vi "Single VLC DisplayN.vi"() -> ()   [LabVIEW 2017]
uses:
  <vilib>/Utility/miscctls.llb/LVRectTypeDef.ctl
  VideoWindowsCommand.ctl
  Video Command type.ctl
  <vilib>/Utility/config.llb/NI_LVConfig.lvlib
  System.Windows.Forms
panel:
  in  "Camera 1":refnum<k24>(container)
  in  "Hide":bool
  in  "Connect":bool
  in  "Cameras":string[](array[string])=["http://admin:pass1234@192.168.1.64/ISAPI/Streaming/channels/102/httpPreview", "http://admin:pass1234@192.168.1.65/ISAPI/Streaming/channels/102/httpPreview", "//192.168.1.119:4747/video"]
  in  "Address":string
  out "InstanceNumber":i32
  in  "Video Feed":enum16{"Camera 1", "Camera2", "Mobile"}(ring)=enum."Camera2"
  in  "Exit":bool
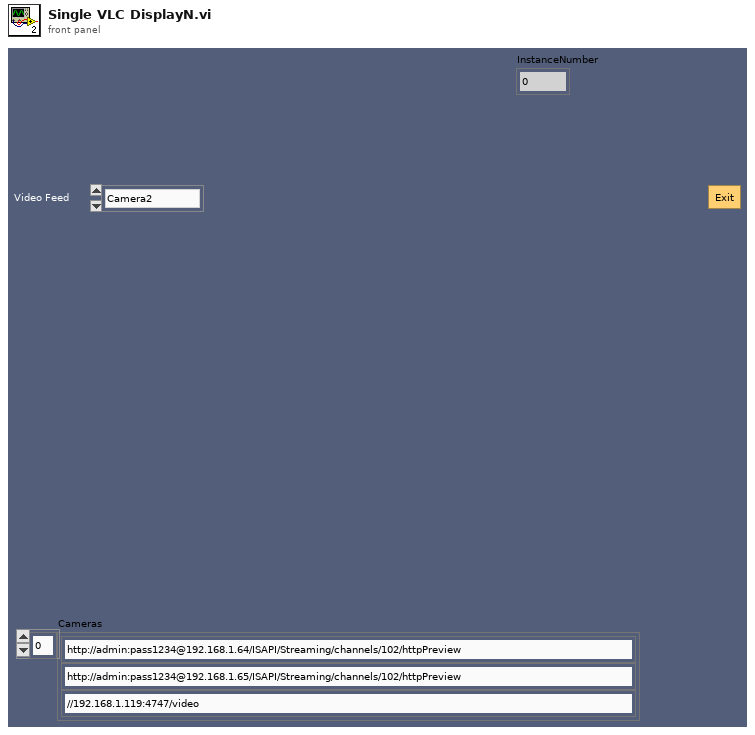
[diagram p1: front panel]
types:
  T1 = typedef "LVRectTypeDef.ctl" = cluster{"Left":i16, "Top":i16, "Right":i16, "Bottom":i16}
  T2 = typedef "NI_LVConfig.lvlib/Config Data RefNum.ctl" = refnum<k1>
  T3 = typedef "VideoWindowsCommand.ctl" = cluster{"Position":cluster{"Right":i32, "Bottom":i32}, "Action":T4, "Camera Addresses":cluster{"Camera 1":string, "Camera 2":string, "Mobile":string}}
  T4 = typedef "Video Command type.ctl" = enum16{"Show", "Hide", "Exit", "Kick"}
  T5 = cluster{"Camera 1":string, "Camera 2":string, "Mobile":string}
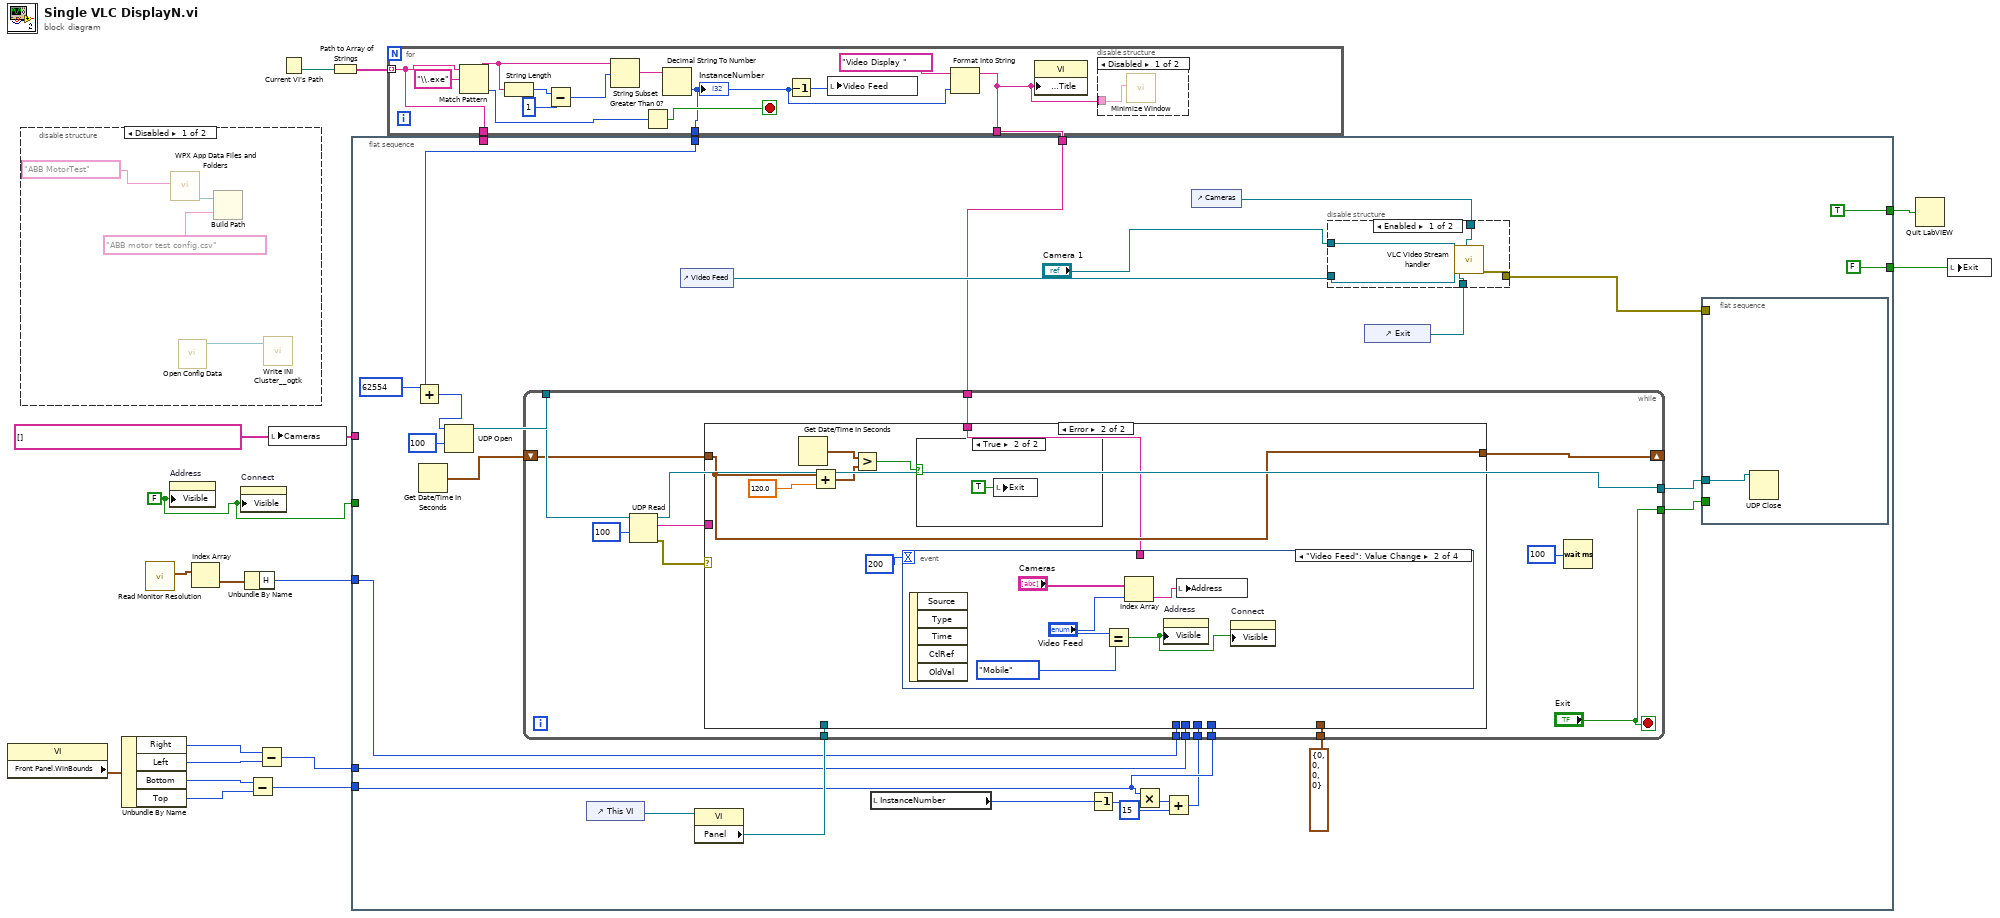
[diagram p0: block diagram]
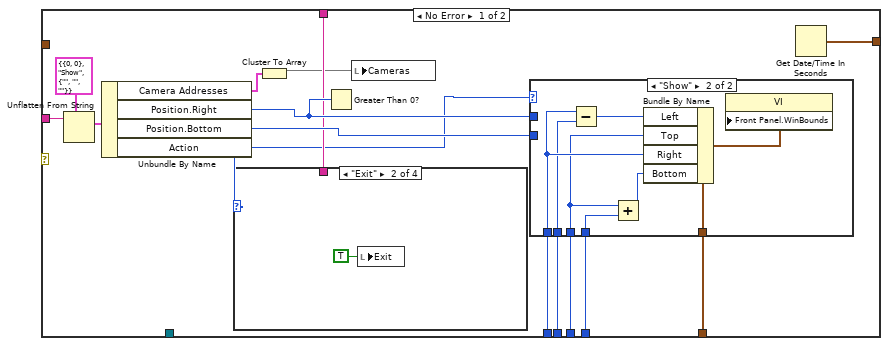
[diagram p4: hidden frame]
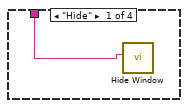
[diagram p5: hidden frame]
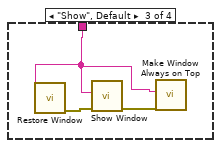
[diagram p6: hidden frame]
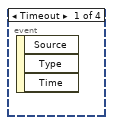
[diagram p10: hidden frame]
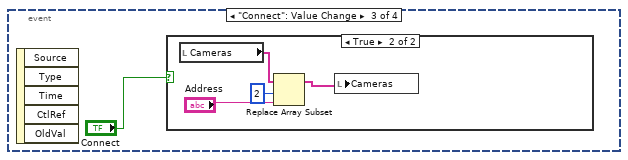
[diagram p11: hidden frame]
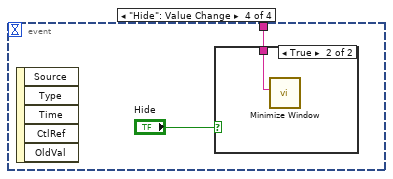
[diagram p13: hidden frame]
diagram:
  w1 = string[] [] ("Cameras")
  w4 = FALSE ("Visible")
  n1 = property class="VI"() -> ("Front Panel.WinBounds"=w12:T1)  [unwired: 2 in, 2 out]
  n2 = disable-structure shown="Disabled" {
    frame Disabled {
      n3 = call "WPX App Data Files and Folders.vi"("ApplicationName"="ABB MotorTest") -> ("DataFolder"=w20:path)  [unwired: 7 in, 3 out]
      n4 = call <vilib>:"Open Config Data.vi"() -> ("refnum"=w23:T2)  [unwired: 9 in, 2 out]
      n5 = Build Path(base path=w20, name or relative path="ABB motor test config.csv") -> ()  [unwired: 1 out]
      n6 = call <userlib>:"Write INI Cluster__ogtk.vi"("refnum"=w23) -> ()  [unwired: 9 in, 2 out]
    }
    frame Enabled {
    }
  }
  n7 = Unbundle By Name(w12) -> ("Right"=w9:i16, "Left"=w8:i16, "Bottom"=w11:i16, "Top"=w10:i16)
  n8 = call "Read Monitor Resolution.vi"() -> ("Monitor Resolution"=w14:cluster{"V":i16, "H":i16}[])  [unwired: 9 in, 2 out]
  n9 = property on="Address" class="Str"("Visible"=w4) -> ()  [unwired: 2 in, 2 out]
  n10 = Index Array(array=w14) -> (element=w13:cluster{"V":i16, "H":i16})  [unwired: 1 in]
  n11 = property on="Connect" class="Bool"("Visible"=w4) -> ()  [unwired: 2 in, 2 out]
  n12 = Unbundle By Name(w13) -> ("H"=w7:i16)
  n13 = Subtract(x=w11, y=w10) -> (x-y=w5:i16)
  n14 = Subtract(x=w9, y=w8) -> (x-y=w6:i16)
  n15 = local write "Cameras"(w1) -> ()
  n16 = Current VI's Path() -> (path=w19:path)
  n17 = Path to Array of Strings(0:w19) -> (2:w18:string[])  [unwired: 1 out]
  n18 = flat-sequence {
    tunnel: w17 -> [w40]
    tunnel: w16 -> [_]
    tunnel: w15 -> [w38]
    tunnel: w7 -> [w37]
    tunnel: w6 -> [w36]
    tunnel: w5 -> [w32]
    tunnel: w4 -> [_]
    tunnel: [TRUE] -> w3
    tunnel: [FALSE ("Exit")] -> w2
    tunnel: w1 -> [_]
    frame #0 {
      n19 = Add(x=w40, y=u16 62554 ("port")) -> (x+y=w39:i32)
      n20 = Get Date/Time In Seconds() -> (seconds since 1Jan1904=w25:timestamp)
      n21 = UDP Open(9:100 ("timeout ms (25000)"), 11:w39) -> (port=w47:refnum<k16>)  [unwired: 3 in, 2 out]
      n22 = control-ref of="This VI"() -> (w46:refnum<vi>)
      n23 = control-ref of="Video Feed"() -> (w50:refnum<vi>)
      n24 = property class="VI"(reference=w46) -> ("Panel"=w45:refnum<vi>)  [unwired: 1 in, 2 out]
      n25 = local read "InstanceNumber"() -> (w34:i32)
      n26 = Decrement(x=w34) -> (x-1=w33:i32)
      n27 = Multiply(x=w32, y=w33) -> (x*y=w30:i32)
      n28 = Add(x=w30, y=15) -> (x+y=w29:i32)
      n29 = while {
        tunnel: ["Exit"] -> w48
        tunnel: w47 -> [w66]
        tunnel: w45 -> [w62]
        tunnel: [w61] -> w44
        tunnel: w38 -> [w60]
        tunnel: w37 -> [w59]
        tunnel: w36 -> [w58]
        tunnel: T1 {"Left"=0, "Top"=0, "Right"=0, "Bottom"=0} ("Front Panel Window:Window Bounds") -> [w57]
        tunnel: w29 -> [w56]
        tunnel: w32 -> [w55]
        shift-right: [w53] -> _
        shift-left: w25 -> [w52]
        stop <- "Exit" stop-if-true
        n30 = UDP Read(connection ID=w66, timeout ms (25000)=100) -> (data out=w63:string, error out=w64:errorcluster, 3:w61:refnum<k16>)  [unwired: 2 in, 2 out]
        n31 = case shown="Error" w64 {
          tunnel: w63 -> [w82 _]
          tunnel: w62 -> [_ _]
          tunnel: w60 -> [w72 w96]
          tunnel: w59 -> [w77 _]
          tunnel: w58 -> [w76 _]
          tunnel: w57 -> [w75 _]
          tunnel: w56 -> [w74 _]
          tunnel: w55 -> [w73 _]
          tunnel: [w70 w97] -> w53
          tunnel: w52 -> [_ w97]
          frame No Error {
            n32 = Unflatten From String(type=T3 {"Position"={"Right"=0, "Bottom"=0}, "Action"=enum."Show", "Camera Addresses"={"Camera 1"="", "Camera 2"="", "Mobile"=""}}, binary string=w82) -> (value=w80:T3)  [unwired: 3 in, 2 out]
            n33 = Unbundle By Name(w80) -> ("Camera Addresses"=w69:T5, "Position.Right"=w78:i32, "Position.Bottom"=w79:i32, "Action"=w71:T4)
            n34 = case shown="\"Exit\"" w71 {
              tunnel: w72 -> [w83 _ w86 _]
              frame "Hide" {
                n35 = call "Hide Window.vi"("window name (\"\")"=w83) -> ()  [unwired: 5 in, 2 out]
              }
              frame "Exit" {
                n36 = local write "Exit"(TRUE ("Exit")) -> ()
              }
              frame "Show", Default {
                n37 = call "Restore Window.vi"("window name  (\"\")"=w86) -> ("error out"=w85:errorcluster)  [unwired: 5 in, 1 out]
                n38 = call "Show Window.vi"("error in (no error)"=w85, "window name (\"\")"=w86) -> ("error out"=w87:errorcluster)  [unwired: 4 in, 1 out]
                n39 = call "Make Window Always on Top.vi"("error in (no error)"=w87, "window name (\"\")"=w86) -> ()  [unwired: 4 in, 2 out]
              }
              frame "Kick" {
              }
            }
            n40 = Cluster To Array(cluster=w69) -> (array=w68:string[])
            n41 = Greater Than 0?(x=w78) -> ()  [unwired: 1 out]
            n42 = local write "Cameras"(w68) -> ()
            n43 = case shown="\"Show\"" w71 {
              tunnel: w79 -> [_ _]
              tunnel: w78 -> [_ _]
              tunnel: w77 -> [_ w92]
              tunnel: w76 -> [_ w91]
              tunnel: w75 -> [_ w90]
              tunnel: w74 -> [_ w89]
              tunnel: w73 -> [_ w88]
              frame "Hide", Default {
              }
              frame "Show" {
                n44 = Subtract(x=w92, y=w91) -> (x-y=w94:i16)
                n45 = Add(x=w89, y=w88) -> (x+y=w93:i32)
                n46 = Bundle By Name(cluster=w90, "Left"=w94, "Top"=w89, "Right"=w92, "Bottom"=w93) -> (w95:T1)
                n47 = property class="VI"("Front Panel.WinBounds"=w95) -> ()  [unwired: 2 in, 2 out]
              }
            }
            n48 = Get Date/Time In Seconds() -> (seconds since 1Jan1904=w70:timestamp)
          }
          frame Error {
            n49 = Get Date/Time In Seconds() -> (seconds since 1Jan1904=w101:timestamp)
            n50 = Add(x=w97, y=120.0) -> (x+y=w99:timestamp)
            n51 = Greater?(x=w101, y=w99) -> (0:w98:bool)
            n52 = event shown="[1] \"Video Feed\": Value Change" {
              selector: _ -> [_ _ _ _]
              dyn-events: _ -> [_ _ _ _]
              timeout: 200 -> [_ _ _ _]
              tunnel: w96 -> [_ _ _ w114]
              event Timeout {
                n53 = event-data() -> ()  [unwired: 1 in, 3 out]
              }
              event "Video Feed": Value Change {
                n54 = event-data() -> ()  [unwired: 1 in, 5 out]
                n55 = Equal?(x="Video Feed", y=enum16{"Camera 1", "Camera2", "Mobile"}."Mobile") -> (x = y?=w107:bool)
                n56 = Index Array(array="Cameras", index="Video Feed") -> (element=w104:string)
                n57 = property on="Address" class="Str"("Visible"=w107) -> ()  [unwired: 2 in, 2 out]
                n58 = local write "Address"(w104) -> ()
                n59 = property on="Connect" class="Bool"("Visible"=w107) -> ()  [unwired: 2 in, 2 out]
              }
              event "Connect": Value Change {
                n60 = event-data() -> ()  [unwired: 1 in, 5 out]
                n61 = case shown="True" "Connect" {
                  frame False {
                  }
                  frame True {
                    n62 = local read "Cameras"() -> (w113:string[])
                    n63 = Replace Array Subset(array=w113, new element="Address", index=2) -> (w112:string[])
                    n64 = local write "Cameras"(w112) -> ()
                  }
                }
              }
              event "Hide": Value Change {
                n65 = event-data() -> ()  [unwired: 1 in, 5 out]
                n66 = case shown="True" "Hide" {
                  tunnel: w114 -> [_ w116]
                  frame False {
                  }
                  frame True {
                    n67 = call "Minimize Window.vi"("window name  (\"\")"=w116) -> ()  [unwired: 5 in, 2 out]
                  }
                }
              }
            }
            n68 = case shown="True" w98 {
              frame False {
              }
              frame True {
                n69 = local write "Exit"(TRUE ("Exit")) -> ()
              }
            }
          }
        }
        n70 = Wait (ms)(milliseconds to wait=u32 100) -> ()  [unwired: 1 out]
      }
      n71 = control-ref of="Cameras"() -> (w31:refnum<vi>)
      n72 = control-ref of="Exit"() -> (w42:refnum<vi>)
      n73 = disable-structure shown="Enabled" {
        disable-tunnel: "Camera 1" -> [w118 _]
        disable-tunnel: w50 -> [w121 _]
        disable-tunnel: [w120 _] -> w49
        disable-tunnel: w42 -> [w119 _]
        disable-tunnel: w31 -> [w117 _]
        frame Enabled {
          n74 = call "VLC Video Stream handler.vi"("CameraArray"=w117, "Exit"=w119, "Video Feed 2"=w121, "Camera 1"=w118) -> ("error out"=w120:errorcluster)  [unwired: 7 in]
        }
        frame Disabled {
        }
      }
      n75 = flat-sequence {
        tunnel: w49 -> [_]
        tunnel: w48 -> [_]
        tunnel: w44 -> [w51]
        frame #0 {
          n76 = UDP Close(connection ID=w51) -> ()  [unwired: 1 in, 2 out]
        }
      }
    }
  }
  n77 = for {
    tunnel: w18 -> [w125] mode=indexing
    tunnel: [w123] -> w17
    tunnel: [w125] -> w16
    tunnel: [w122] -> w15
    stop <- w127 stop-if-true
    n78 = Match Pattern(string=w125, regular expression="\\.exe") -> (before substring=w133:string, offset past match=w128:i32)  [unwired: 1 in, 2 out]
    n79 = String Length(string=w133) -> (length=w132:i32)
    n80 = Subtract(x=w132, y=1) -> (x-y=w130:i32)
    n81 = String Subset(string=w133, offset (0)=w130) -> (substring=w129:string)  [unwired: 1 in]
    n82 = Greater Than 0?(x=w128) -> (x > 0?=w127:bool)
    n83 = Decimal String To Number(string=w129) -> (number=w123:i32)  [unwired: 2 in, 1 out]
    "InstanceNumber" <- w123
    n84 = Decrement(x=w123) -> (x-1=w126:i32)
    n85 = local write "Video Feed"(w126) -> ()
    n86 = Format Into String(initial string="Video Display ", w123) -> (resulting string=w122:string)  [unwired: 2 in, 1 out]
    n87 = property class="VI"("Front Panel.Title"=w122) -> ()  [unwired: 2 in, 2 out]
    n88 = disable-structure shown="Disabled" {
      disable-tunnel: w122 -> [w135 _]
      frame Disabled {
        n89 = call "Minimize Window.vi"("window name  (\"\")"=w135) -> ()  [unwired: 5 in, 2 out]
      }
      frame Enabled {
      }
    }
  }
  n90 = Quit LabVIEW(quit? (T)=w3) -> ()
  n91 = local write "Exit"(w2) -> ()
